vi "电导率电极校准.vi"() -> ()   [LabVIEW 2016, in "斯坦道多参数.lvlib"]
uses:
  <vilib>/Utility/miscctls.llb/LVPointTypeDef.ctl
  <vilib>/Analysis/NI_AALBase.lvlib
panel:
  in  "刷新按钮":bool
  out "第二点信号值":dbl
  out "第一点信号值":dbl
  out "通讯状态":string
  out "盐度":dbl caption="盐度测量值" format="%#.2f"
  out "温度":dbl format="%#.2f"
  out "当前信号值":dbl caption="信号值" format="%#.2f"
  in  "校准停止":bool
  in  "校准启动":bool
  out "波形图表":dbl(graph) caption="历史曲线"
  out "第二点校准值":dbl
  out "第一点校准值":dbl
  in  "校准模式":u16(ring)=1 items=["两点校准", "单点校准"]
  out "提示":string
  out "最小值":sgl format="%#.2f"
  out "最大值":sgl format="%#.2f"
  out "mean":dbl caption="均值" format="%#.2f"
  out "standard deviation":dbl caption="标准差" format="%#.2f"
  out "变异系数":dbl format="%#.6f"
  out "标液2":dbl
  out "标液1":dbl
  out "当前读取值":dbl caption="测量值" format="%#.2f"
  out "电极系数":dbl format="%#.6f"
  out "偏移值补偿":dbl caption="电导率偏移修正值" format="%#.2f"
  out "温度补偿系数":dbl format="%#.6f"
  # "电导率电极设定"
  # "ppt"
  # "请选择校准模式:"
  # "℃"
  # "μS/cm"
  # "cm"
  # "-1"
  # "%"
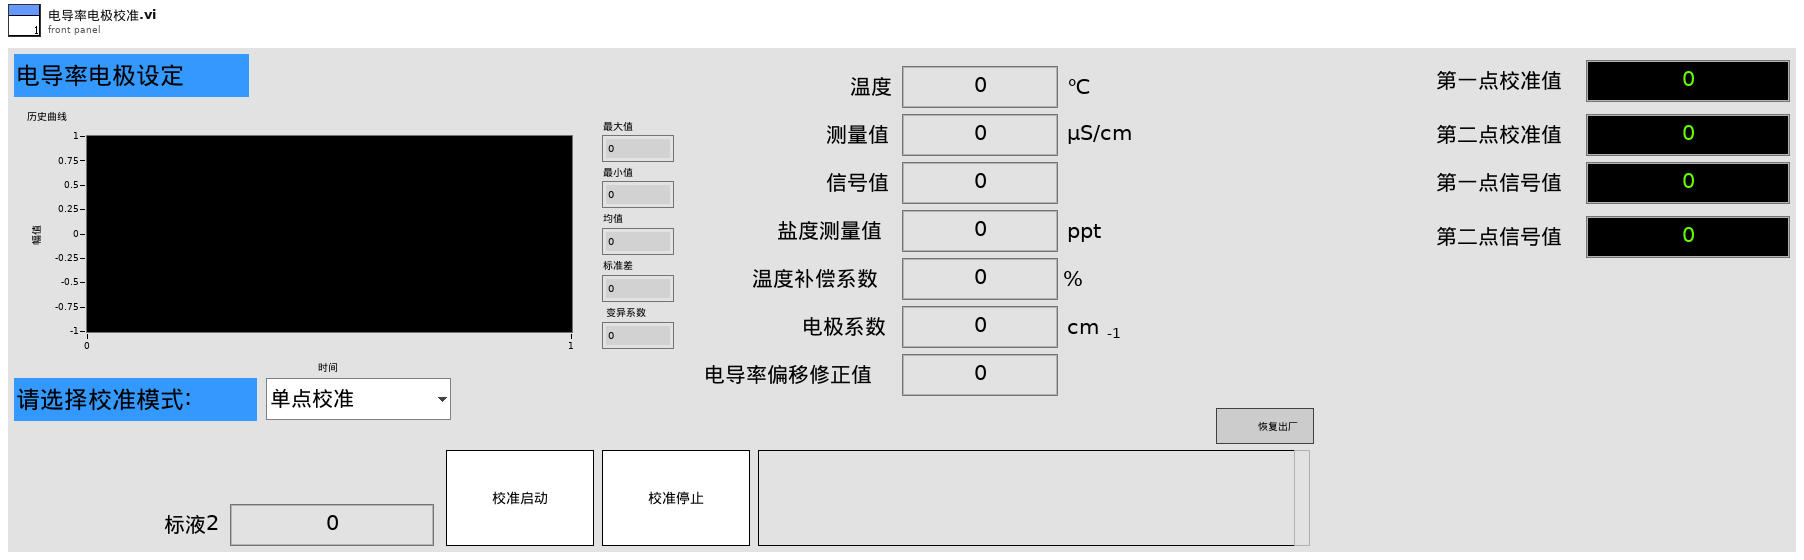
[diagram p1: front panel]
types:
  T1 = typedef "LVPointTypeDef.ctl" = cluster{"Horizontal":i16, "Vertical":i16}
  T2 = cluster{"电极状态标志":u16, "电极型号标志":u16, "电导率测量值":sgl, "温度测量值":sgl, "电导率信号值":sgl, "温度信号值":sgl, "温度补偿系数":sgl, "电导率偏移修正值":sgl, "温度偏移修正值":sgl, "手动温度补偿值":sgl, "电导率电极零点":sgl, "电导率电极斜率":sgl, "命令滤波设定":u16, "温度模式":enum16{"ATC", "MTC"}, "生产批次":u16, "电极序号":u16, "串口地址":u16, "串口波特率":enum16{"9600", "19200", "115200"}, "串口校验位":enum16{"NONE", "ODD", "EVEN"}, "串口停止位":enum16{"1bit", "2bit"}, "第一点标准值":sgl, "第二点标准值":sgl}
  T3 = enum8{"Enabled", "Disabled", "Disabled and Grayed Out"}
  T4 = cluster{"ph":bool, "DO":bool, "Cond":bool, "Turb":bool, "叶绿素a":bool, "藻密度":bool, "ORP":bool}
  T5 = cluster{"温度测量值":sgl, "测量值":sgl, "温度偏移修正值":sgl, "信号值":sgl}
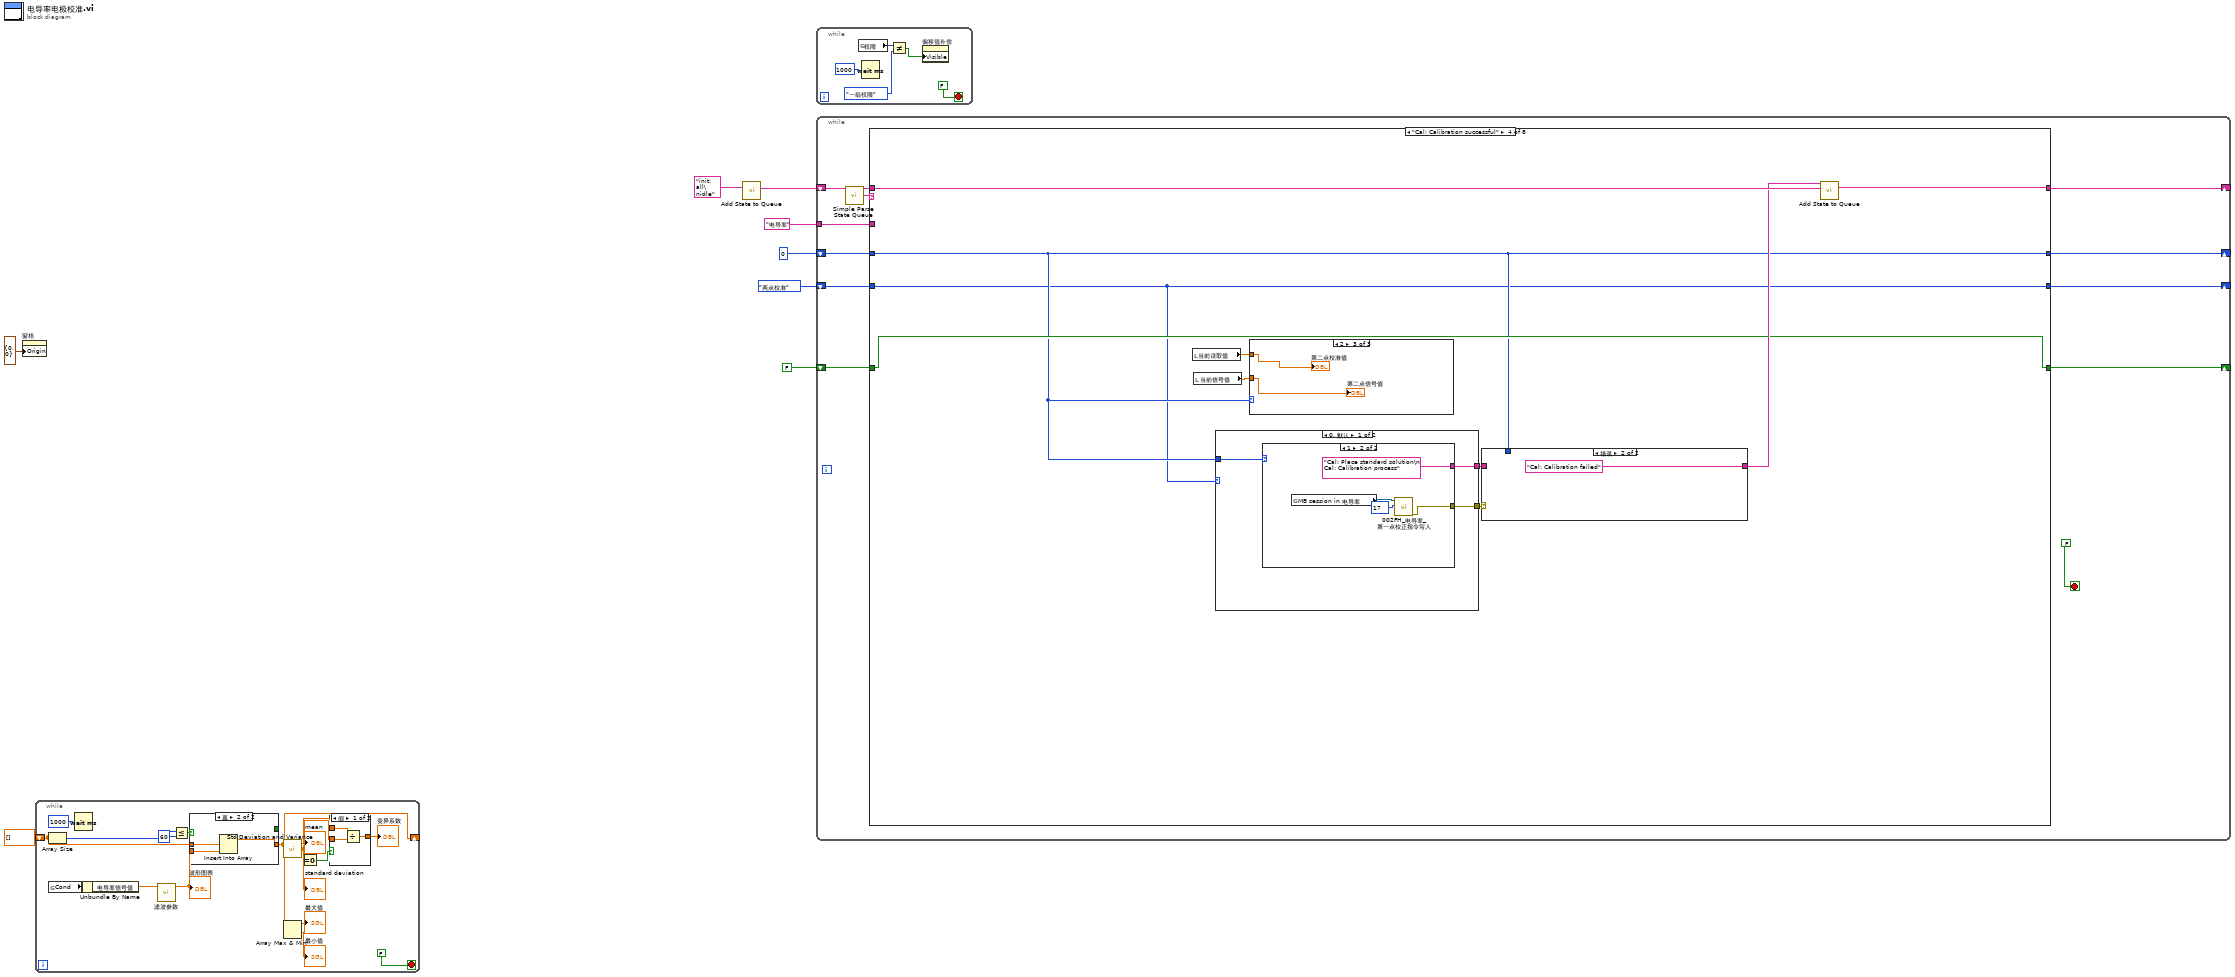
[diagram p0: block diagram]
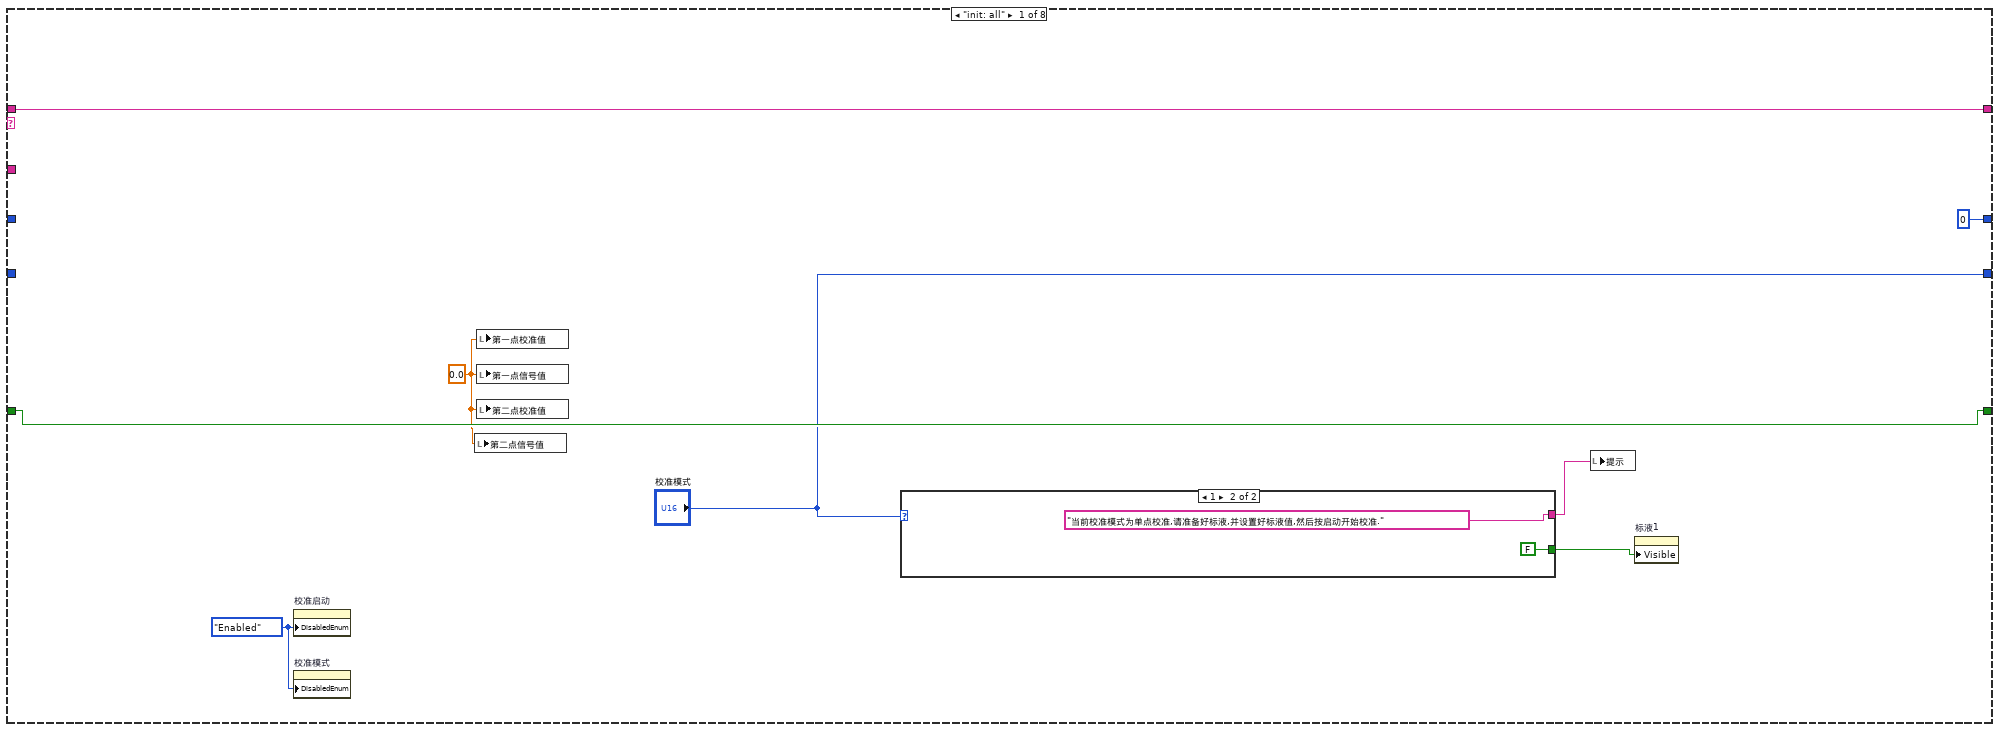
[diagram p2: hidden frame]
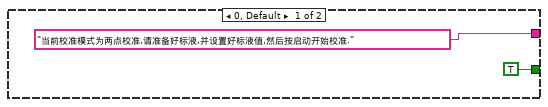
[diagram p3: hidden frame]
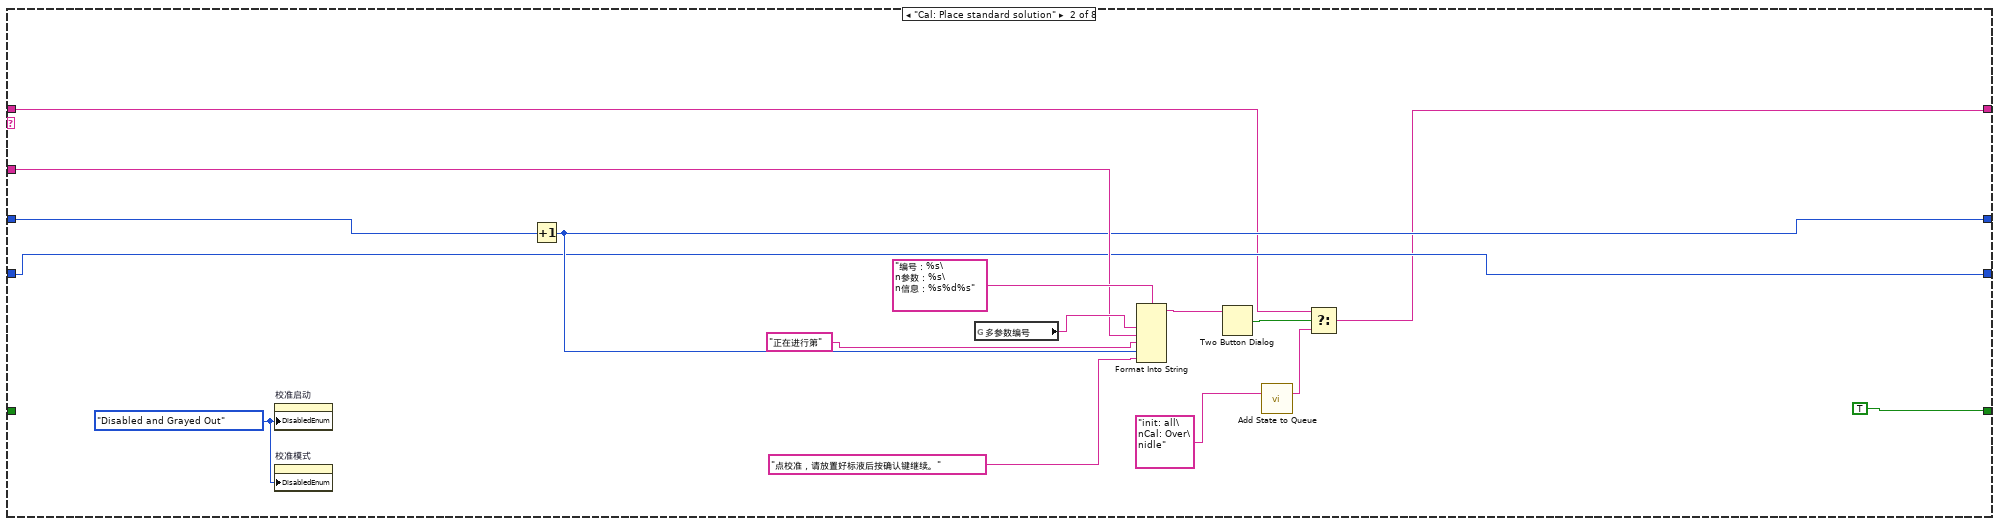
[diagram p4: hidden frame]
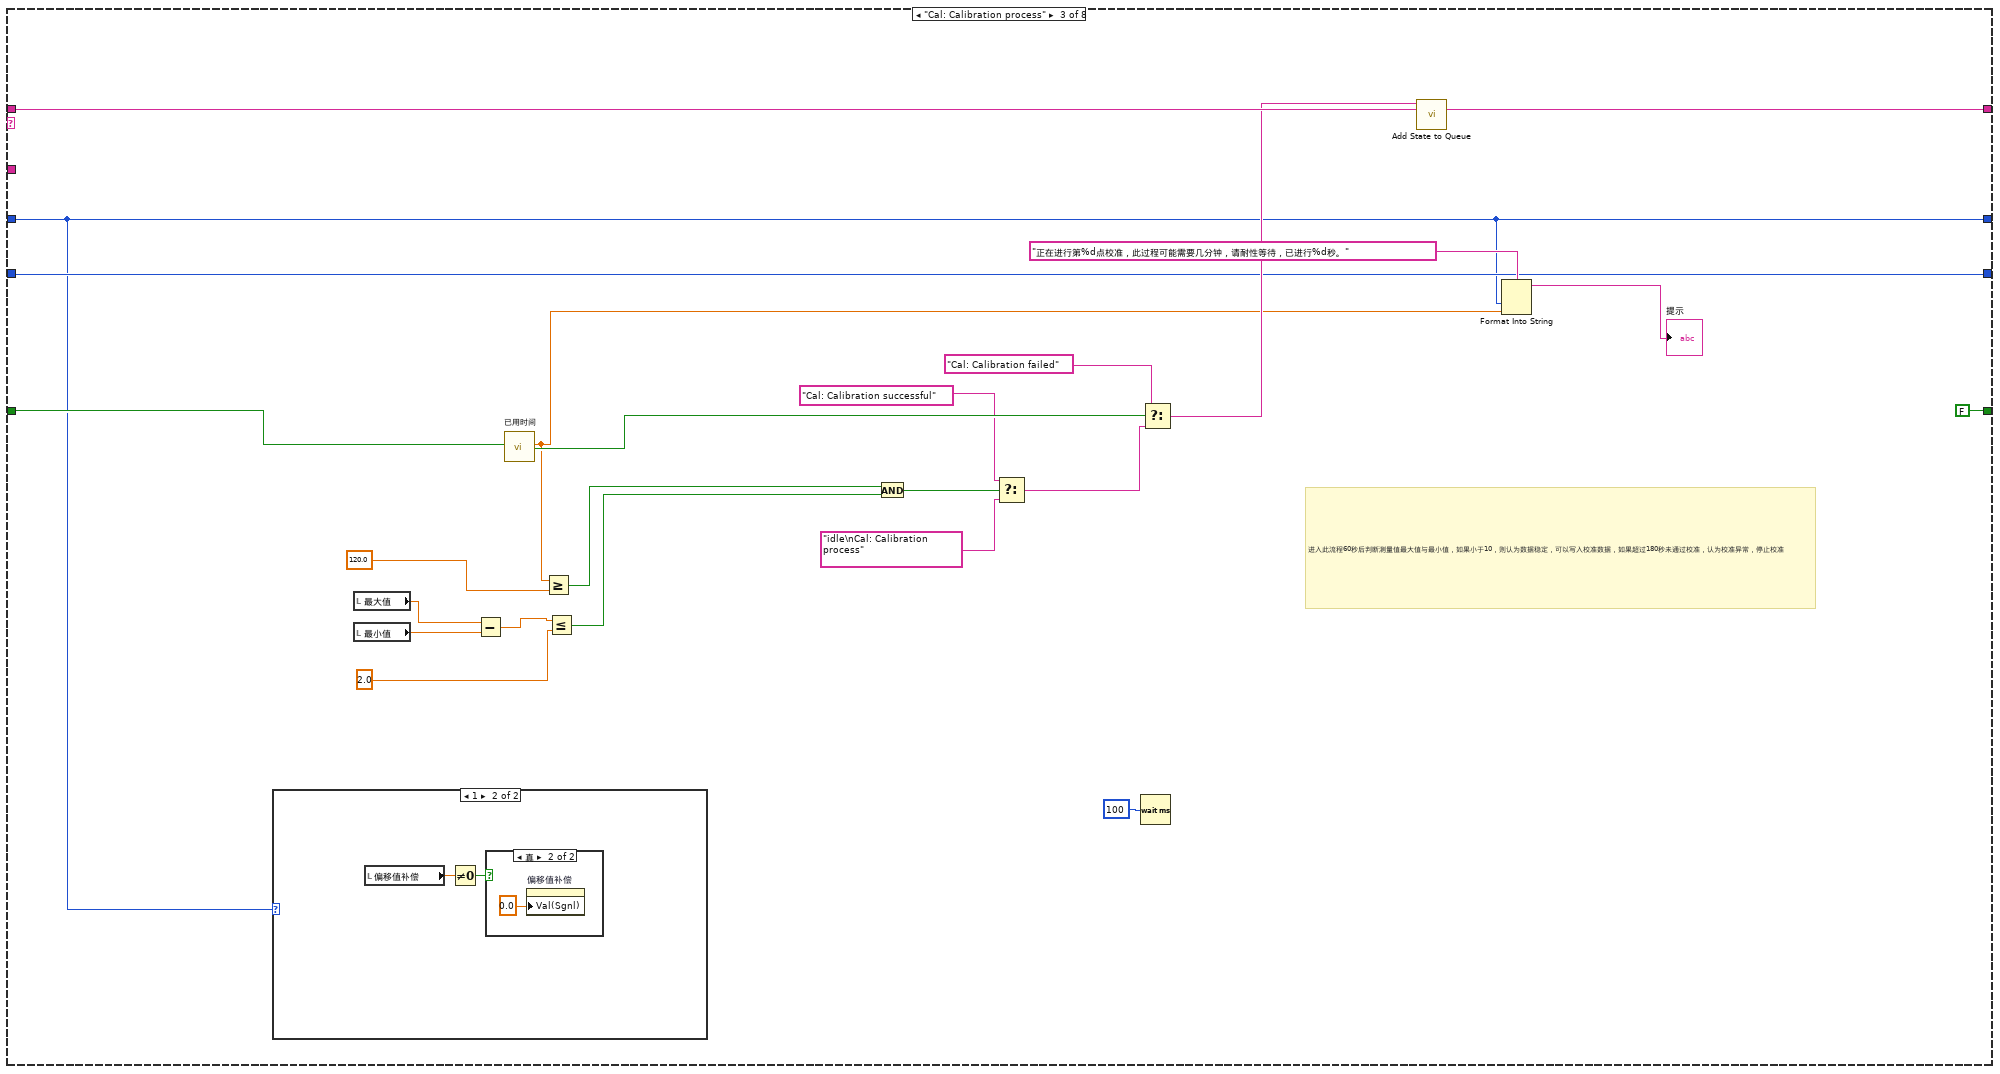
[diagram p5: hidden frame]
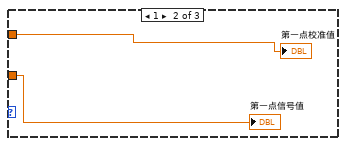
[diagram p9: hidden frame]
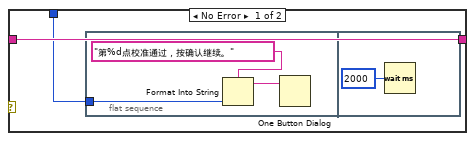
[diagram p10: hidden frame]
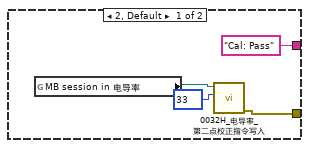
[diagram p11: hidden frame]
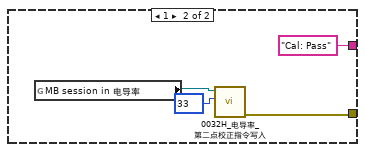
[diagram p12: hidden frame]
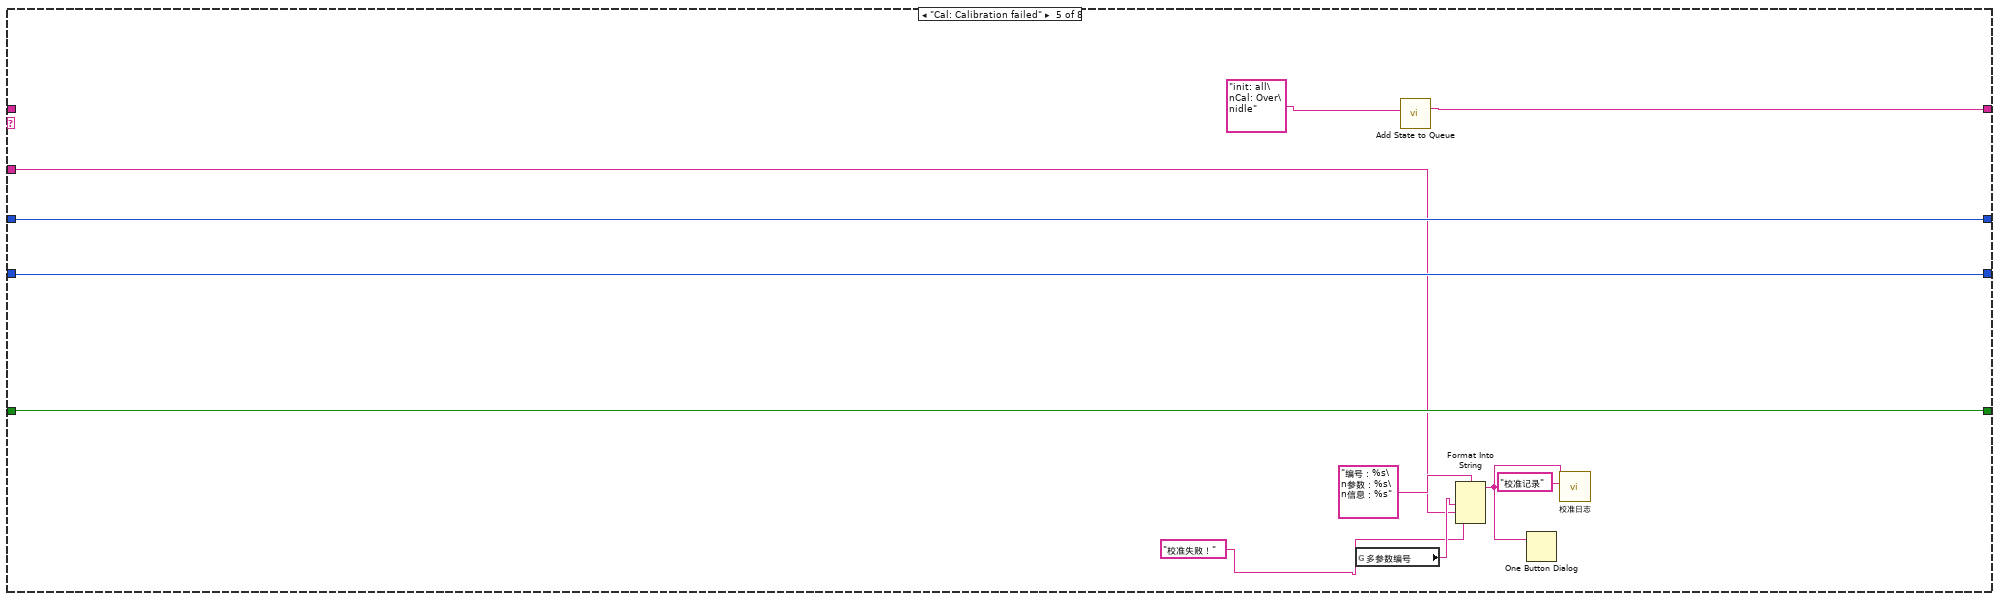
[diagram p13: hidden frame]
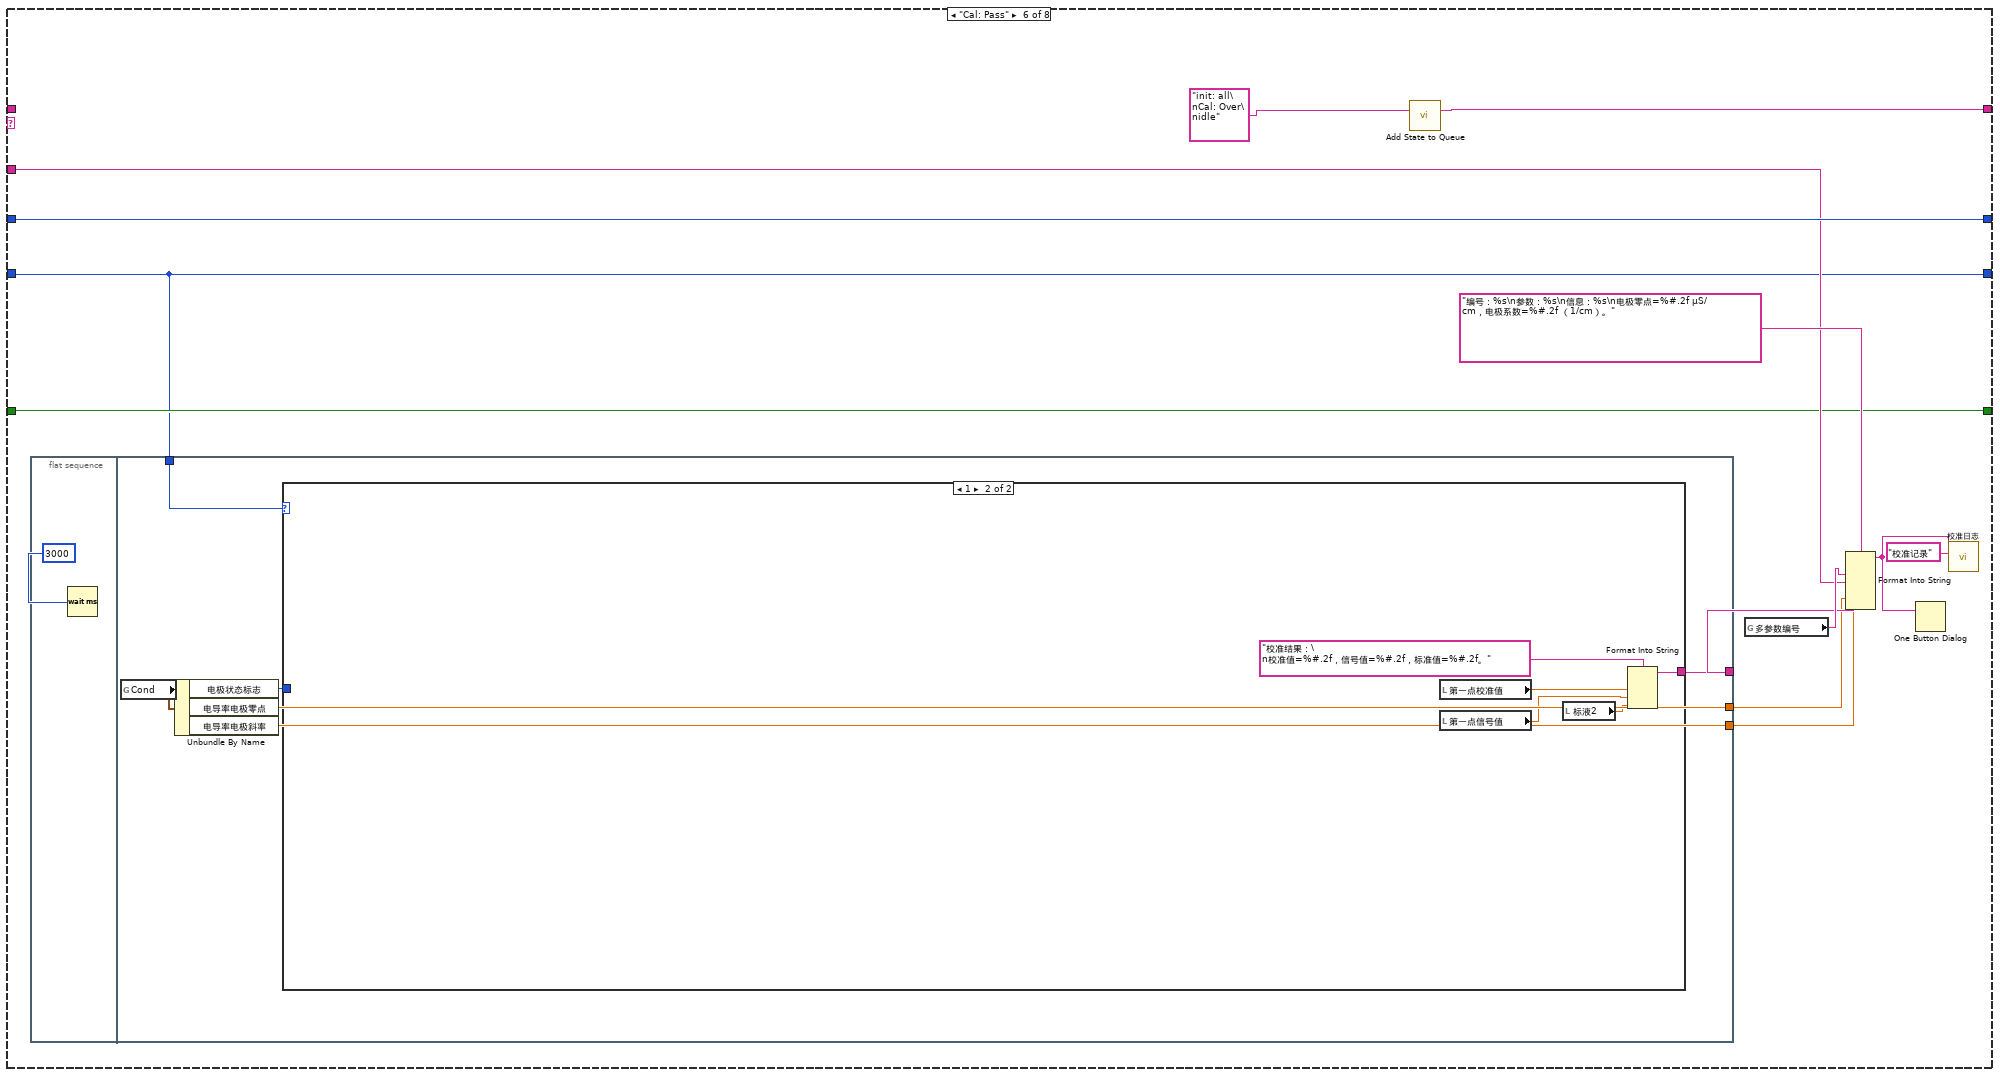
[diagram p14: hidden frame]
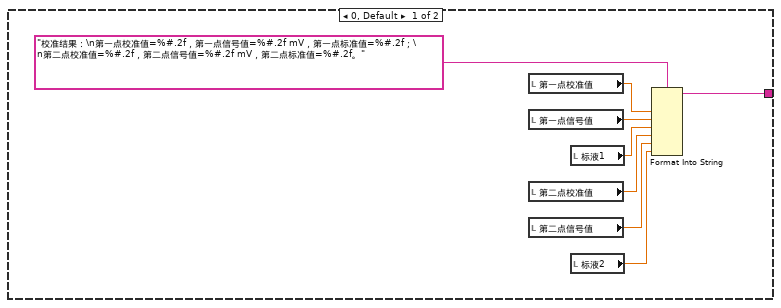
[diagram p15: hidden frame]
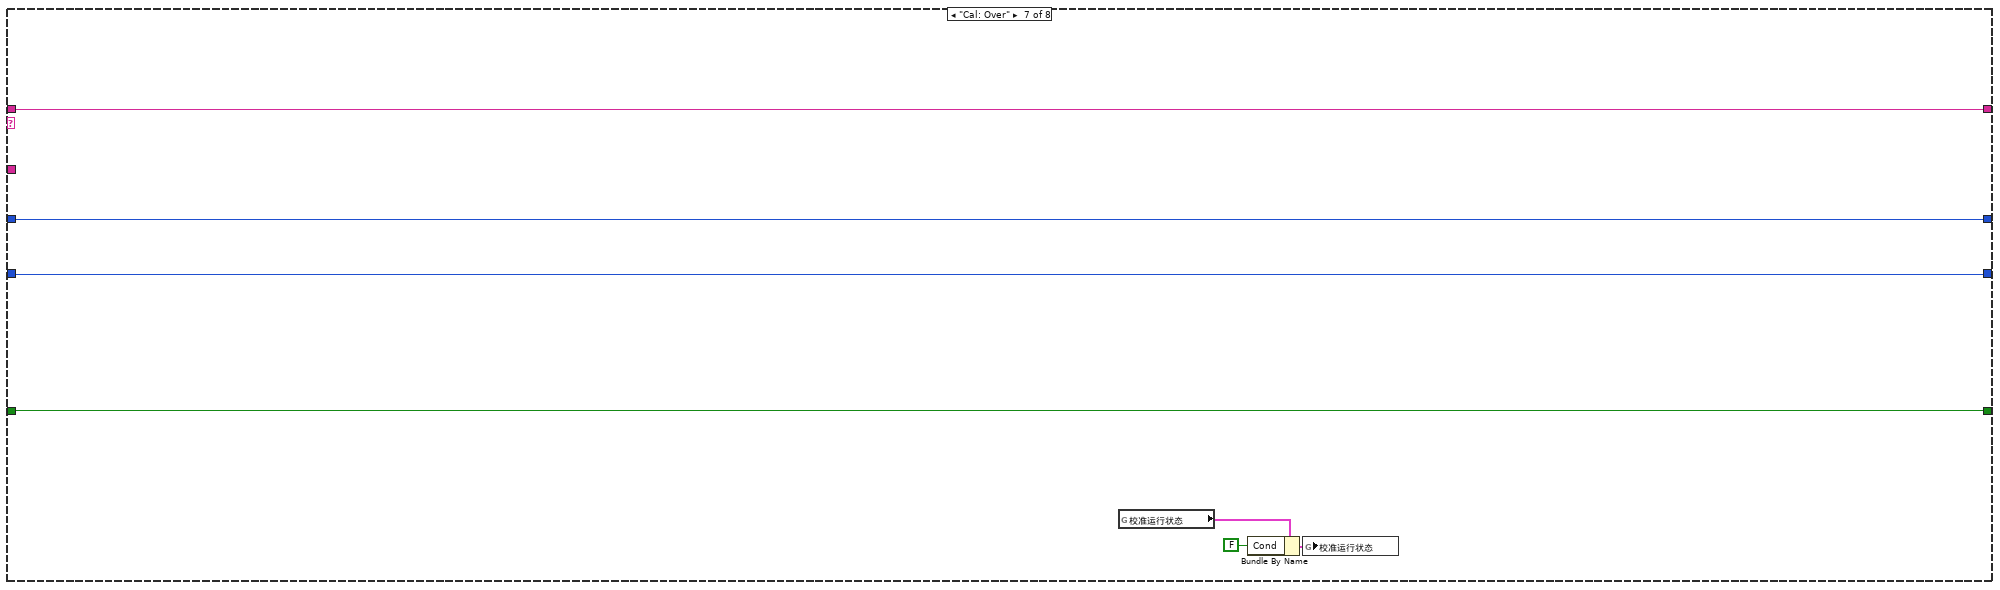
[diagram p16: hidden frame]
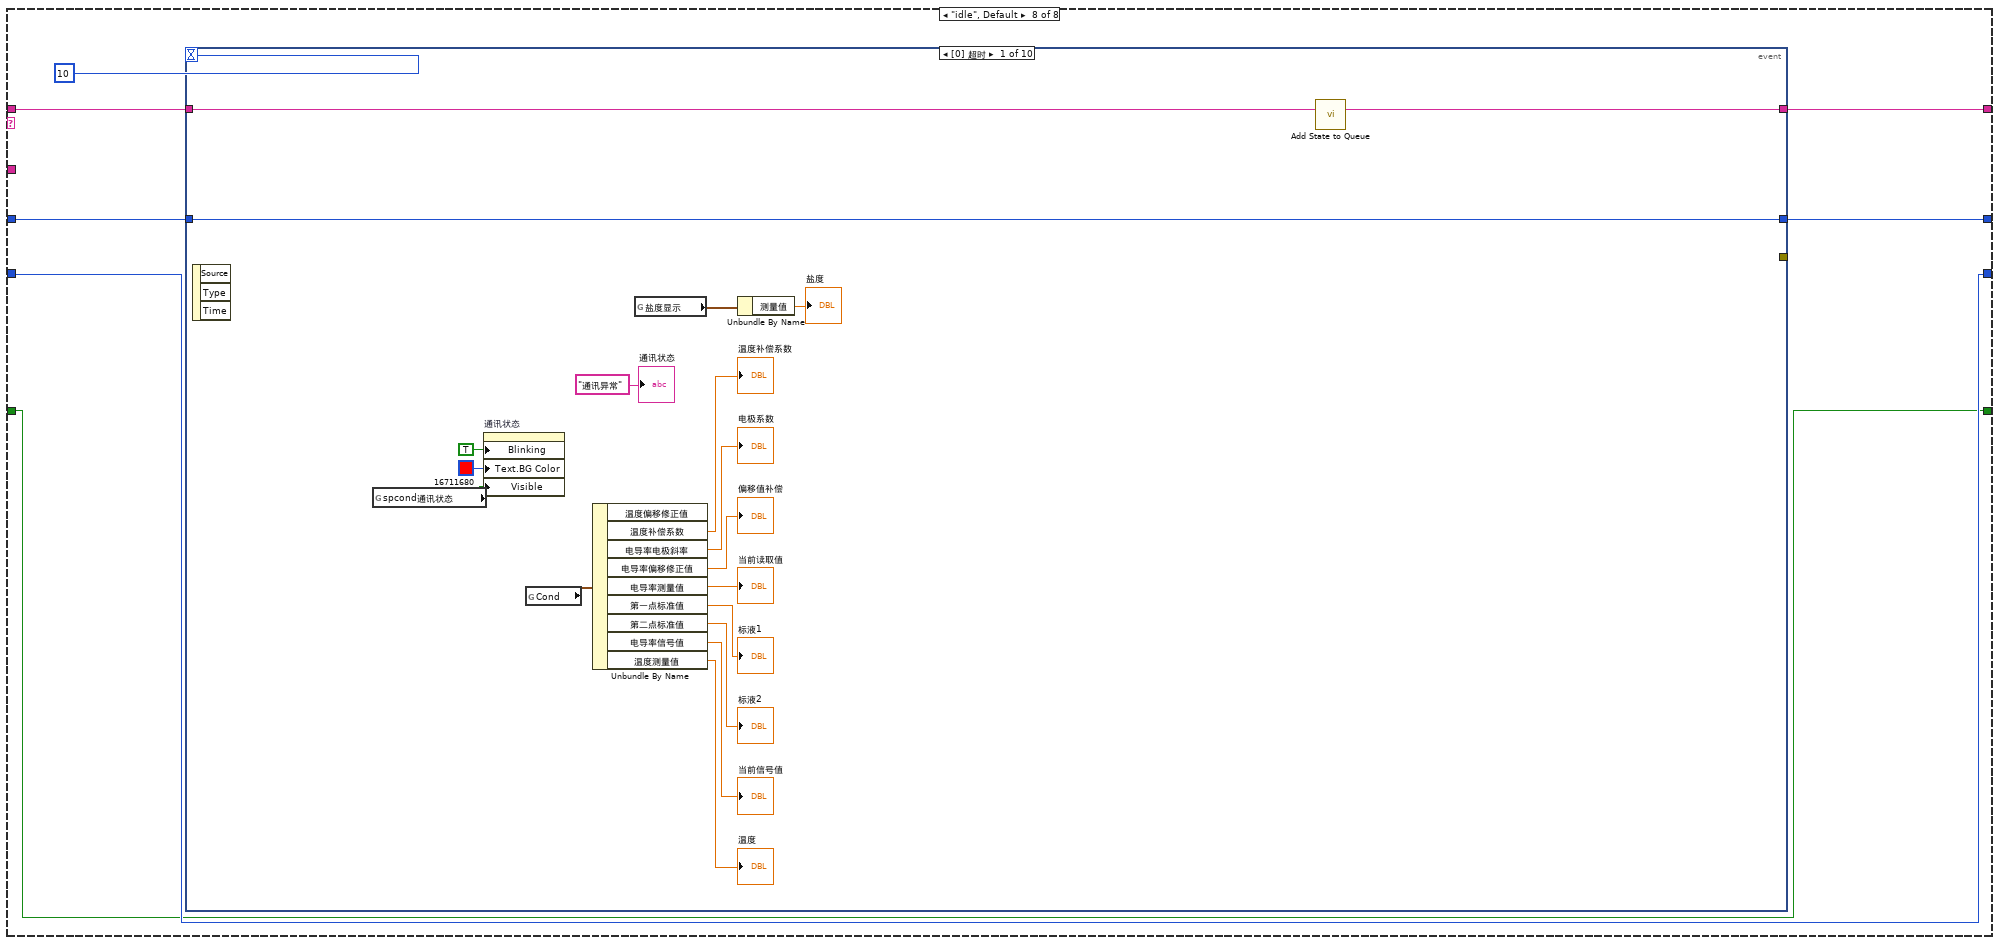
[diagram p17: hidden frame]
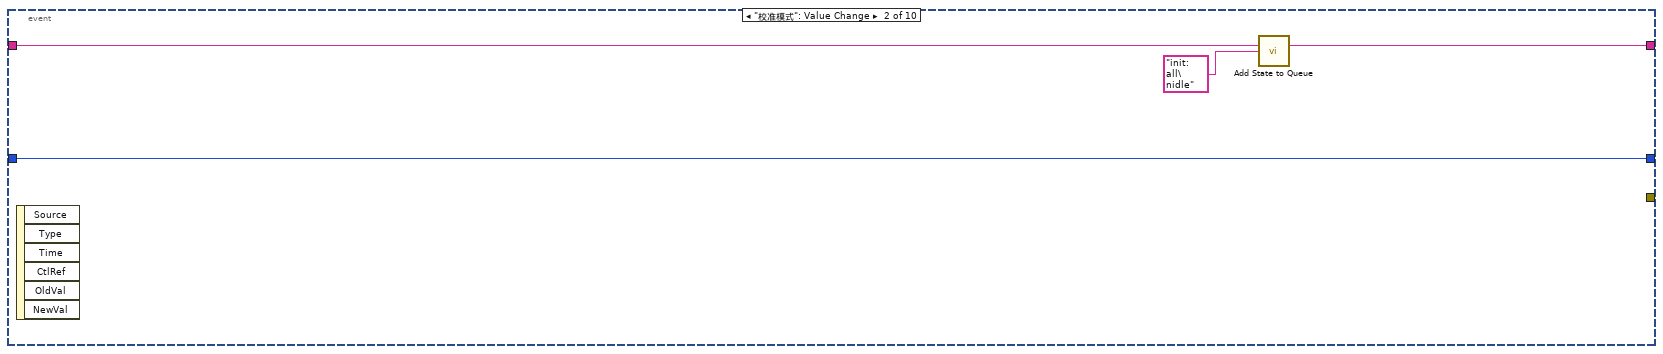
[diagram p18: hidden frame]
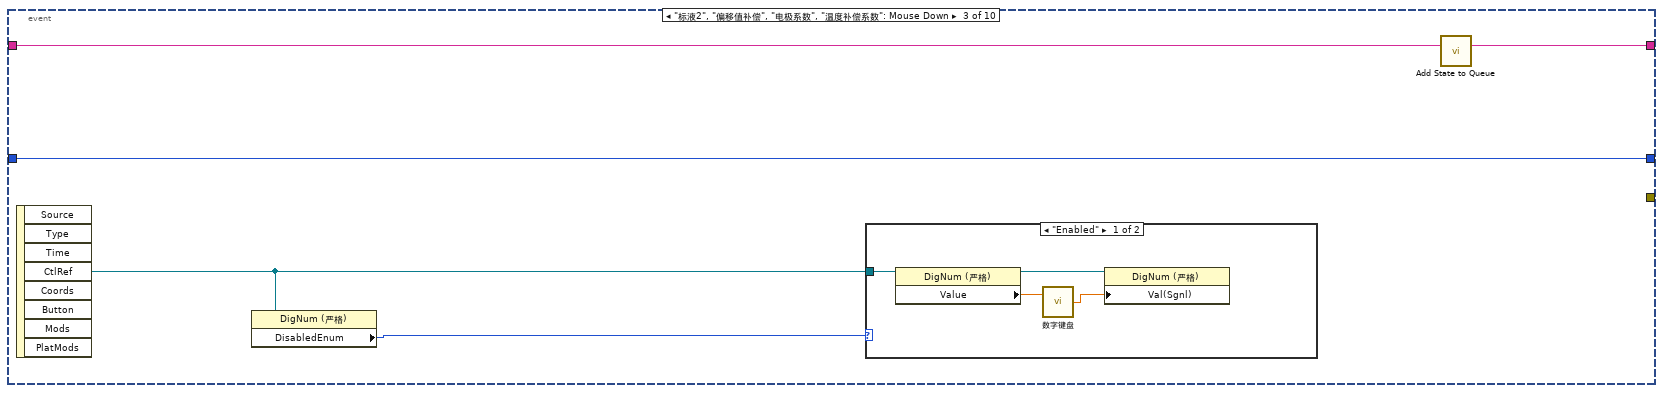
[diagram p19: hidden frame]
diagram:
  n1 = property on="窗格" class="Pane"("Origin"=T1 {"Horizontal"=0, "Vertical"=0} ("原点")) -> ()  [unwired: 2 in, 2 out]
  n2 = while {
    shift-right: [w13] -> _
    shift-left: sgl[] [] -> [w20]
    stop <- FALSE stop-if-true
    n3 = Array Size(array=w20) -> (size(s)=w22:i32)
    n4 = global read "国弘过程全局变量.vi" "Cond"() -> (w14:T2)
    n5 = Wait (ms)(milliseconds to wait=u32 1000 ("等待时间（毫秒）")) -> ()  [unwired: 1 out]
    n6 = Unbundle By Name(w14) -> ("电导率信号值"=w10:sgl)
    n7 = call "滤波参数.vi"("x"=w10) -> ("mode"=w9:dbl)  [unwired: 10 in]
    "波形图表" <- w9
    n8 = Less Or Equal?(x=w22, y=60) -> (x <= y?=w21:bool)
    n9 = case shown="真" w21 {
      tunnel: w20 -> [w33 w36]
      tunnel: w9 -> [w31 w35]
      tunnel: [w29 w34] -> w13
      tunnel: [TRUE _] -> _
      frame False {
        n10 = Replace Array Subset(array=w33, new element=w31) -> (w32:sgl[])  [unwired: 1 in]
        n11 = Rotate 1D Array(1:w32, 2:-1 ("n")) -> (0:w29:sgl[])
      }
      frame True {
        n12 = Insert Into Array(array=w36, new element=w35) -> (w34:sgl[])  [unwired: 1 in]
      }
    }
    n13 = call <vilib>:"Std Deviation and Variance.vi"("X"=w13) -> ("mean"=w18:dbl, "standard deviation"=w17:dbl)  [unwired: 1 in, 1 out]
    "mean" <- w18
    "standard deviation" <- w17
    n14 = Array Max & Min(array=w13) -> (max value=→"最大值":sgl, min value=→"最小值":sgl)  [unwired: 2 out]
    n15 = Equal To 0?(x=w18) -> (x = 0?=w19:bool)
    n16 = case shown="假" w19 {
      tunnel: w17 -> [w27 _]
      tunnel: [w26 _] -> w16
      tunnel: w18 -> [w25 _]
      frame False {
        n17 = Divide(x=w27, y=w25) -> (x/y=w26:dbl)
      }
      frame True {
      }
    }
    "变异系数" <- w16
  }
  n18 = call "Add State to Queue.vi"("State(s) In (\"\")"="init: all\nidle" ("State(s) In (\"\")")) -> ("States Out"=w5:string)  [unwired: 14 in]
  n19 = while {
    stop <- FALSE stop-if-true
    n20 = global read "多参数全局变量.vi" "权限"() -> (w40:enum16{"一级权限", "二级权限", "三级权限"})
    n21 = Wait (ms)(milliseconds to wait=u32 1000 ("等待时间（毫秒）")) -> ()  [unwired: 1 out]
    n22 = Not Equal?(x=w40, y=enum16{"一级权限", "二级权限", "三级权限"}."一级权限") -> (x != y?=w38:bool)
    n23 = property on="偏移值补偿" class="DigNum (严格)"("Visible"=w38) -> ()  [unwired: 2 in, 2 out]
  }
  n24 = while {
    shift-right: [w49] -> _
    shift-left: w5 -> [w53]
    shift-right: [w46] -> _
    shift-left: 0 -> [w48]
    tunnel: "电导率" ("State(s) In (\"\")") -> [w47]
    shift-right: [w44] -> _
    shift-left: enum16{"两点校准", "单点校准"}."两点校准" ("校准模式") -> [w45]
    shift-right: [w42] -> _
    shift-left: FALSE -> [w43]
    stop <- FALSE stop-if-true
    n25 = call "Simple Parse State Queue.vi"("State Queue"=w53) -> ("Remain States"=w50:string, "Next State"=w51:string)  [unwired: 13 in]
    n26 = case shown="\"Cal: Calibration successful\"" w51 {
      tunnel: w50 -> [w61 w69 w100 w116 _ _ w195 w202]
      tunnel: [w61 w68 w99 w115 w152 w159 w195 w201] -> w49
      tunnel: w48 -> [_ w77 w84 w110 w155 w168 w194 w199]
      tunnel: w47 -> [_ w78 _ _ w146 w164 _ _]
      tunnel: [0 w75 w84 w110 w155 w168 w194 w200] -> w46
      tunnel: w45 -> [_ w74 w85 w109 w154 w160 w193 w198]
      tunnel: ["校准模式" w74 w85 w109 w154 w160 w193 w198] -> w44
      tunnel: w43 -> [w58 _ w87 w111 w153 w163 w192 w196]
      tunnel: [w58 TRUE FALSE w111 w153 w163 w192 w196] -> w42
      frame "init: all" {
        w56 = T3."Enabled" ("禁用")
        w55 = 0.0 ("第一点校准值")
        n27 = property on="校准启动" class="Bool"("DisabledEnum"=w56) -> ()  [unwired: 2 in, 2 out]
        n28 = property on="校准模式" class="Ring (严格)"("DisabledEnum"=w56) -> ()  [unwired: 2 in, 2 out]
        n29 = local write "第二点信号值"(w55) -> ()
        n30 = local write "第一点校准值"(w55) -> ()
        n31 = local write "第一点信号值"(w55) -> ()
        n32 = local write "第二点校准值"(w55) -> ()
        n33 = case shown="1" "校准模式" {
          tunnel: ["当前校准模式为两点校准,请准备好标液,并设置好标液值,然后按启动开始校准." ("提示") "当前校准模式为单点校准,请准备好标液,并设置好标液值,然后按启动开始校准." ("提示")] -> w60
          tunnel: [TRUE ("可见") FALSE ("可见")] -> w54
          frame 0, Default {
          }
          frame 1 {
          }
        }
        n34 = local write "提示"(w60) -> ()
        n35 = property on="标液1" class="DigNum (严格)"("Visible"=w54) -> ()  [unwired: 2 in, 2 out]
      }
      frame "Cal: Place standard solution" {
        w67 = T3."Disabled and Grayed Out" ("禁用")
        n36 = property on="校准启动" class="Bool"("DisabledEnum"=w67) -> ()  [unwired: 2 in, 2 out]
        n37 = property on="校准模式" class="Ring (严格)"("DisabledEnum"=w67) -> ()  [unwired: 2 in, 2 out]
        n38 = Increment(x=w77) -> (x+1=w75:i32)
        n39 = global read "多参数全局变量.vi" "多参数编号"() -> (w80:string)
        n40 = Format Into String(format string="编号：%s\n参数：%s\n信息：%s%d%s" ("格式字符串"), w80, w78, "正在进行第" ("消息"), w75, "点校准，请放置好标液后按确认键继续。" ("消息")) -> (resulting string=w72:string)  [unwired: 2 in, 1 out]
        n41 = Two Button Dialog(message=w72) -> (T button?=w71:bool)  [unwired: 2 in]
        n42 = call "Add State to Queue.vi"("State(s) In (\"\")"="init: all\nCal: Over\nidle" ("State(s) In (\"\")")) -> ("States Out"=w70:string)  [unwired: 14 in]
        n43 = Select(t=w69, s=w71, f=w70) -> (s? t:f=w68:string)
      }
      frame "Cal: Calibration process" {
        # "进入此流程60秒后判断测量值最大值与最小值，如果小于10，则认为数据稳定，可以写入校准数据，如果超过180秒未通过校准，认为校准异常，停止校准"
        n44 = case shown="1" w84 {
          frame 0, Default {
          }
          frame 1 {
            n45 = local read "偏移值补偿"() -> (w106:dbl)
            n46 = Not Equal To 0?(x=w106) -> (x != 0?=w107:bool)
            n47 = case shown="真" w107 {
              frame False {
              }
              frame True {
                n48 = property on="偏移值补偿" class="DigNum (严格)"("Val(Sgnl)"=0.0 ("值(信号)")) -> ()  [unwired: 2 in, 2 out]
              }
            }
          }
        }
        n49 = local read "最大值"() -> (w104:sgl)
        n50 = local read "最小值"() -> (w103:sgl)
        n51 = Subtract(x=w104, y=w103) -> (x-y=w105:sgl)
        n52 = call "已用时间"("Reset"=w87) -> ("Elapsed Time (s)"=w83:dbl, "Time has Elapsed"=w101:bool)  [unwired: 11 in, 6 out]
        n53 = Greater Or Equal?(x=w83, y=120.0) -> (x >= y?=w96:bool)
        n54 = Less Or Equal?(x=w105, y=2.0) -> (x <= y?=w92:bool)
        n55 = And(x=w96, y=w92) -> (x .and. y?=w93:bool)
        n56 = Select(t="Cal: Calibration successful" ("State(s) In (\"\")"), s=w93, f="idle\nCal: Calibration process" ("State(s) In (\"\")")) -> (s? t:f=w91:string)
        n57 = Wait (ms)(milliseconds to wait=u32 100 ("等待时间（毫秒）")) -> ()  [unwired: 1 out]
        n58 = Select(t="Cal: Calibration failed" ("State(s) In (\"\")"), s=w101, f=w91) -> (s? t:f=w90:string)
        n59 = call "Add State to Queue.vi"("State(s) In Front (\"\")"=w90, "State(s) In (\"\")"=w100) -> ("States Out"=w99:string)  [unwired: 13 in]
        n60 = Format Into String(format string="正在进行第%d点校准，此过程可能需要几分钟，请耐性等待，已进行%d秒。" ("格式字符串"), w84, w83) -> (resulting string=→"提示":string)  [unwired: 2 in, 1 out]
      }
      frame "Cal: Calibration successful" {
        n61 = local read "当前读取值"() -> (w112:dbl)
        n62 = local read "当前信号值"() -> (w113:dbl)
        n63 = case shown="0, 默认" w109 {
          tunnel: [w132 w141] -> w118
          tunnel: [w131 "Cal: Pass" ("State(s) In (\"\")")] -> w117
          tunnel: w110 -> [w130 _]
          frame 0, Default {
            n64 = case shown="1" w130 {
              tunnel: [w133 w137] -> w132
              tunnel: ["Cal: Pass" ("State(s) In (\"\")") "Cal: Place standard solution\n Cal: Calibration process" ("State(s) In (\"\")")] -> w131
              frame 2, Default {
                n65 = global read "多参数全局变量.vi" "MB session in 电导率"() -> (w135:refnum<class "MB_Master.lvclass">)
                n66 = call "0032H_电导率_第二点校正指令写入.vi"("数值"=u16 33, "MB session in"=w135) -> ("error out"=w133:errorcluster)  [unwired: 8 in, 1 out]
              }
              frame 1 {
                n67 = global read "多参数全局变量.vi" "MB session in 电导率"() -> (w139:refnum<class "MB_Master.lvclass">)
                n68 = call "002FH_电导率_第一点校正指令写入.vi"("数值"=u16 17, "MB session in"=w139) -> ("error out"=w137:errorcluster)  [unwired: 8 in, 1 out]
              }
            }
          }
          frame 1 {
            n69 = global read "多参数全局变量.vi" "MB session in 电导率"() -> (w143:refnum<class "MB_Master.lvclass">)
            n70 = call "0032H_电导率_第二点校正指令写入.vi"("数值"=u16 33, "MB session in"=w143) -> ("error out"=w141:errorcluster)  [unwired: 8 in, 1 out]
          }
        }
        n71 = case shown="2" w110 {
          tunnel: w113 -> [_ w120 w122]
          tunnel: w112 -> [_ w119 w121]
          frame 0, Default {
          }
          frame 1 {
            "第一点信号值" <- w120
            "第一点校准值" <- w119
          }
          frame 2 {
            "第二点信号值" <- w122
            "第二点校准值" <- w121
          }
        }
        n72 = case shown="错误" w118 {
          tunnel: w117 -> [w124 _]
          tunnel: [w124 "Cal: Calibration failed" ("State(s) In (\"\")")] -> w114
          tunnel: w110 -> [w123 _]
          frame No Error {
            n73 = flat-sequence {
              tunnel: w123 -> [w125]
              frame #0 {
                n74 = Format Into String(format string="第%d点校准通过，按确认继续。" ("格式字符串"), w125) -> (resulting string=w127:string)  [unwired: 2 in, 1 out]
                n75 = One Button Dialog(message=w127) -> ()  [unwired: 1 in, 1 out]
              }
              frame #1 {
                n76 = Wait (ms)(milliseconds to wait=u32 2000 ("等待时间（毫秒）")) -> ()  [unwired: 1 out]
              }
            }
          }
          frame Error {
          }
        }
        n77 = call "Add State to Queue.vi"("State(s) In Front (\"\")"=w114, "State(s) In (\"\")"=w116) -> ("States Out"=w115:string)  [unwired: 13 in]
      }
      frame "Cal: Calibration failed" {
        n78 = global read "多参数全局变量.vi" "多参数编号"() -> (w149:string)
        n79 = call "Add State to Queue.vi"("State(s) In (\"\")"="init: all\nCal: Over\nidle" ("State(s) In (\"\")")) -> ("States Out"=w152:string)  [unwired: 14 in]
        n80 = Format Into String(format string="编号：%s\n参数：%s\n信息：%s" ("格式字符串"), w149, w146, "校准失败！" ("消息")) -> (resulting string=w148:string)  [unwired: 2 in, 1 out]
        n81 = One Button Dialog(message=w148) -> ()  [unwired: 1 in, 1 out]
        n82 = call "校准日志.vi"("table"="校准记录", "日志信息"=w148) -> ()  [unwired: 9 in, 1 out]
      }
      frame "Cal: Pass" {
        n83 = flat-sequence {
          tunnel: [w173] -> w161
          tunnel: w160 -> [w172]
          tunnel: [w171] -> w158
          tunnel: [w170] -> w157
          frame #0 {
            n84 = Wait (ms)(milliseconds to wait=u32 3000 ("等待时间（毫秒）")) -> ()  [unwired: 1 out]
          }
          frame #1 {
            n85 = global read "国弘过程全局变量.vi" "Cond"() -> (w174:T2)
            n86 = Unbundle By Name(w174) -> ("电极状态标志"=w175:u16, "电导率电极零点"=w171:sgl, "电导率电极斜率"=w170:sgl)
            n87 = case shown="1" w172 {
              tunnel: [w183 w188] -> w173
              tunnel: w175 -> [_ _]
              frame 0, Default {
                n88 = local read "第一点校准值"() -> (w181:dbl)
                n89 = local read "第一点信号值"() -> (w182:dbl)
                n90 = local read "第二点校准值"() -> (w178:dbl)
                n91 = local read "第二点信号值"() -> (w177:dbl)
                n92 = local read "标液1"() -> (w179:dbl)
                n93 = local read "标液2"() -> (w176:dbl)
                n94 = Format Into String(format string="校准结果：\n第一点校准值=%#.2f，第一点信号值=%#.2f mV，第一点标准值=%#.2f；\n第二点校准值=%#.2f，第二点信号值=%#.2f mV，第二点标准值=%#.2f。" ("提示"), w181, w182, w179, w178, w177, w176) -> (resulting string=w183:string)  [unwired: 2 in, 1 out]
              }
              frame 1 {
                n95 = local read "第一点校准值"() -> (w187:dbl)
                n96 = local read "第一点信号值"() -> (w185:dbl)
                n97 = local read "标液2"() -> (w184:dbl)
                n98 = Format Into String(format string="校准结果：\n校准值=%#.2f，信号值=%#.2f，标准值=%#.2f。" ("提示"), w187, w185, w184) -> (resulting string=w188:string)  [unwired: 2 in, 1 out]
              }
            }
          }
        }
        n99 = call "Add State to Queue.vi"("State(s) In (\"\")"="init: all\nCal: Over\nidle" ("State(s) In (\"\")")) -> ("States Out"=w159:string)  [unwired: 14 in]
        n100 = global read "多参数全局变量.vi" "多参数编号"() -> (w165:string)
        n101 = Format Into String(format string="编号：%s\n参数：%s\n信息：%s\n电极零点=%#.2f μS/cm，电极系数=%#.2f （1/cm）。" ("格式字符串"), w165, w164, w161, w158, w157) -> (resulting string=w162:string)  [unwired: 2 in, 1 out]
        n102 = One Button Dialog(message=w162) -> ()  [unwired: 1 in, 1 out]
        n103 = call "校准日志.vi"("table"="校准记录", "日志信息"=w162) -> ()  [unwired: 9 in, 1 out]
      }
      frame "Cal: Over" {
        n104 = global read "多参数全局变量.vi" "校准运行状态"() -> (w190:T4)
        n105 = Bundle By Name(cluster=w190, "Cond"=FALSE) -> (w191:T4)
        n106 = global write "多参数全局变量.vi" "校准运行状态"(w191) -> ()
      }
      frame "idle", Default {
        n107 = event shown="[0] 超时" {
          selector: _ -> [_ _ _ _ _ _ _ _ _ _]
          dyn-events: _ -> [_ _ _ _ _ _ _ _ _ _]
          timeout: 10 -> [_ _ _ _ _ _ _ _ _ _]
          tunnel: [_ _ _ w235 w243 w247 w252 _ _ _] -> _
          tunnel: w202 -> [w220 w224 w227 w234 w240 w251 w257 w262 w271 _]
          tunnel: [w219 w223 w228 w238 w241 w250 w256 w261 w270 w273] -> w201
          tunnel: [w218 w221 w229 w239 w242 w249 w255 w260 w268 w274] -> w200
          tunnel: w199 -> [w218 w221 w229 w239 w242 w249 w255 w260 w268 w274]
          event Timeout {
            n108 = event-data() -> ()  [unwired: 1 in, 3 out]
            n109 = global read "多参数全局变量.vi" "spcond通讯状态"() -> (w216:bool)
            n110 = property on="通讯状态" class="Str"("Blinking"=TRUE ("闪烁"), "Text.BG Color"=u32 16711680, "Visible"=w216) -> ()  [unwired: 2 in, 2 out]
            n111 = global read "国弘过程全局变量.vi" "Cond"() -> (w203:T2)
            n112 = Unbundle By Name(w203) -> ("温度补偿系数"=→"温度补偿系数":sgl, "电导率电极斜率"=→"电极系数":sgl, "电导率偏移修正值"=→"偏移值补偿":sgl, "电导率测量值"=→"当前读取值":sgl, "第一点标准值"=→"标液1":sgl, "第二点标准值"=→"标液2":sgl, "电导率信号值"=→"当前信号值":sgl, "温度测量值"=→"温度":sgl)  [unwired: 1 out]
            n113 = global read "多参数全局变量.vi" "盐度显示"() -> (w212:T5)
            n114 = Unbundle By Name(w212) -> ("测量值"=→"盐度":sgl)
            n115 = call "Add State to Queue.vi"("State(s) In (\"\")"=w220) -> ("States Out"=w219:string)  [unwired: 14 in]
            "通讯状态" <- "通讯异常" ("当前串口")
          }
          event "校准模式": Value Change {
            n116 = event-data() -> ()  [unwired: 1 in, 6 out]
            n117 = call "Add State to Queue.vi"("State(s) In (\"\")"=w224, "State(s) At Back (\"\")"="init: all\nidle" ("State(s) In (\"\")")) -> ("States Out"=w223:string)  [unwired: 13 in]
          }
          event "标液2", "偏移值补偿", "电极系数", "温度补偿系数": Mouse Down {
            n118 = event-data() -> ("CtlRef"=w226:refnum<vi>)  [unwired: 1 in, 7 out]
            n119 = property class="DigNum (严格)"(reference=w226) -> ("DisabledEnum"=w225:T3)  [unwired: 1 in, 2 out]
            n120 = case shown="\"Enabled\"" w225 {
              tunnel: w226 -> [w233 _]
              frame "Enabled" {
                n121 = property class="DigNum (严格)"(reference=w233) -> (reference out=w230:refnum<vi>, "Value"=w231:dbl)  [unwired: 1 in, 1 out]
                n122 = call "数字键盘.vi"("OldNumber"=w231) -> ("NewNumber"=w232:dbl)  [unwired: 1 in]
                n123 = property class="DigNum (严格)"(reference=w230, "Val(Sgnl)"=w232) -> ()  [unwired: 1 in, 2 out]
              }
              frame "Disabled", Default {
              }
            }
            n124 = call "Add State to Queue.vi"("State(s) In (\"\")"=w227) -> ("States Out"=w228:string)  [unwired: 14 in]
          }
          event "标液2": Value Change {
            n125 = event-data() -> ("NewVal"=w236:dbl)  [unwired: 1 in, 5 out]
            n126 = global read "多参数全局变量.vi" "MB session in 电导率"() -> (w237:refnum<class "MB_Master.lvclass">)
            n127 = call "0033H_电导率_第二点标准值写入.vi"("数值"=w236, "MB session in"=w237) -> ("error out"=w235:errorcluster)  [unwired: 8 in, 1 out]
            n128 = call "Add State to Queue.vi"("State(s) In (\"\")"=w234) -> ("States Out"=w238:string)  [unwired: 14 in]
          }
          event "电极系数": Value Change {
            n129 = event-data() -> ("NewVal"=w244:dbl)  [unwired: 1 in, 5 out]
            n130 = global read "多参数全局变量.vi" "MB session in 电导率"() -> (w245:refnum<class "MB_Master.lvclass">)
            n131 = call "0014H_电导率_电极系数写入.vi"("数值"=w244, "MB session in"=w245) -> ("error out"=w243:errorcluster)  [unwired: 8 in, 1 out]
            n132 = call "Add State to Queue.vi"("State(s) In (\"\")"=w240) -> ("States Out"=w241:string)  [unwired: 14 in]
          }
          event "偏移值补偿": Value Change {
            n133 = event-data() -> ("NewVal"=w246:dbl)  [unwired: 1 in, 5 out]
            n134 = global read "多参数全局变量.vi" "MB session in 电导率"() -> (w248:refnum<class "MB_Master.lvclass">)
            n135 = call "000CH_电导率_电导率偏移修正值写入.vi"("数值"=w246, "MB session in"=w248) -> ("error out"=w247:errorcluster)  [unwired: 8 in, 1 out]
            n136 = call "Add State to Queue.vi"("State(s) In (\"\")"=w251) -> ("States Out"=w250:string)  [unwired: 14 in]
          }
          event "温度补偿系数": Value Change {
            n137 = event-data() -> ("NewVal"=w253:dbl)  [unwired: 1 in, 5 out]
            n138 = global read "多参数全局变量.vi" "MB session in 电导率"() -> (w254:refnum<class "MB_Master.lvclass">)
            n139 = call "000AH_电导率_温度补偿系数写入.vi"("数值"=w253, "MB session in"=w254) -> ("error out"=w252:errorcluster)  [unwired: 8 in, 1 out]
            n140 = call "Add State to Queue.vi"("State(s) In (\"\")"=w257) -> ("States Out"=w256:string)  [unwired: 14 in]
          }
          event "刷新按钮": Value Change {
            n141 = event-data() -> ()  [unwired: 1 in, 6 out]
            n142 = call "Add State to Queue.vi"("State(s) In (\"\")"=w262) -> ("States Out"=w261:string)  [unwired: 14 in]
            n143 = Two Button Dialog(message="请再次确实是否恢复出厂设置！" ("消息")) -> (T button?=w259:bool)  [unwired: 2 in]
            n144 = case shown="真" w259 {
              frame False {
              }
              frame True {
                w263 = u16 33 items=["Factory Reset"=33] ("数值")
                n145 = global read "多参数全局变量.vi" "MB session in 电导率"() -> (w264:refnum<class "MB_Master.lvclass">)
                n146 = call "0026H_电导率_命令寄存器写入.vi"("数值"=w263, "MB session in"=w264) -> ()  [unwired: 8 in, 2 out]
              }
            }
          }
          event "校准启动": Value Change {
            n147 = event-data() -> ()  [unwired: 1 in, 6 out]
            n148 = global read "多参数全局变量.vi" "校准运行状态"() -> (w266:T4)
            n149 = Bundle By Name(cluster=w266, "Cond"=TRUE) -> (w267:T4)
            n150 = global write "多参数全局变量.vi" "校准运行状态"(w267) -> ()
            n151 = call "Add State to Queue.vi"("State(s) In (\"\")"=w271, "State(s) At Back (\"\")"="init: all\nCal: Place standard solution\n Cal: Calibration process\nidle" ("State(s) In (\"\")")) -> ("States Out"=w270:string)  [unwired: 13 in]
          }
          event "校准停止": Value Change {
            n152 = event-data() -> ()  [unwired: 1 in, 6 out]
            n153 = call "Add State to Queue.vi"("State(s) In (\"\")"="init: all\nCal: Over\nidle" ("State(s) In (\"\")")) -> ("States Out"=w273:string)  [unwired: 14 in]
          }
        }
      }
    }
  }
